vi "read_write_DB_Conn_path.vi"(1 "DB Connection Path in":path=path "", 2 "Write?":bool) -> (0 "DB Connection Path":path)   [LabVIEW 2013]
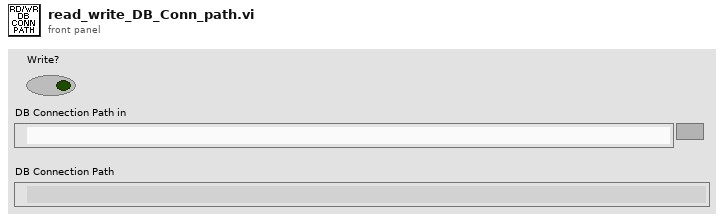
[diagram p1: front panel]
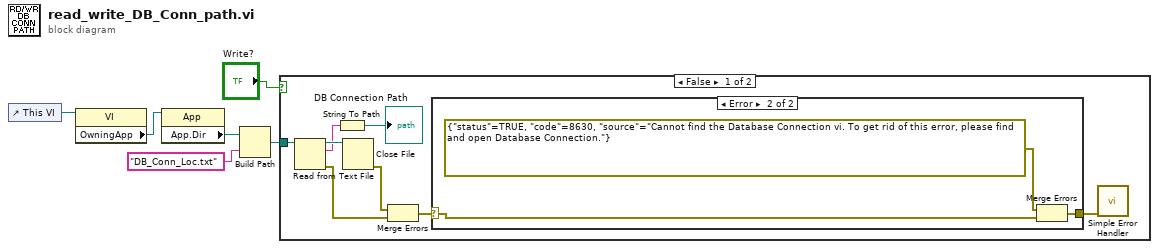
[diagram p0: block diagram]
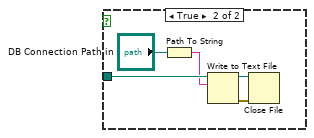
[diagram p3: hidden frame]
diagram:
  n1 = control-ref of="This VI"() -> (w2:refnum<vi>)
  n2 = property class="VI"(reference=w2) -> ("OwningApp"=w3:refnum<vi>)  [unwired: 1 in, 2 out]
  n3 = property class="App"(reference=w3) -> ("App.Dir"=w4:path)  [unwired: 1 in, 2 out]
  n4 = Build Path(base path=w4, name or relative path="DB_Conn_Loc.txt") -> (appended path=w1:path)
  n5 = case shown="False" "Write?" {
    tunnel: w1 -> [w14 w23]
    frame False {
      n6 = Read from Text File(file (use dialog)=w14) -> (refnum out=w13:refnum<file>, text=w12:string, error out=w10:errorcluster)  [unwired: 3 in, 1 out]
      n7 = String To Path(string=w12) -> (path=→"DB Connection Path":path)
      n8 = Close File(refnum=w13) -> (error out=w8:errorcluster)  [unwired: 1 in, 1 out]
      n9 = Merge Errors(w8, w10) -> (w9:errorcluster)
      n10 = case shown="Error" w9 {
        selector: w9 -> [w15 w16]
        tunnel: [w15 w18] -> w7
        frame No Error {
        }
        frame Error {
          n11 = Merge Errors(errorcluster {"status"=TRUE, "code"=8630, "source"="Cannot find the Database Connection vi. To get rid of this error, please find and open Database Connection."} ("error in"), w16) -> (w18:errorcluster)
        }
      }
      n12 = call <vilib>:"Simple Error Handler.vi"("error in (no error)"=w7) -> ()  [unwired: 4 in, 5 out]
    }
    frame True {
      n13 = Path To String(path="DB Connection Path in") -> (string=w21:string)
      n14 = Write to Text File(file (use dialog)=w23, text=w21) -> (refnum out=w20:refnum<file>, error out=w19:errorcluster)  [unwired: 2 in, 1 out]
      n15 = Close File(refnum=w20, error in=w19) -> ()  [unwired: 2 out]
    }
  }
